vi "Filter Cluster Items.vi"(7 "Action":T1, 10 "Filter Str":string, 11 "Display Items":T2[](array[typedef])) -> (3 "Filtered Items":T2[](array[typedef]))   [LabVIEW 2023]
uses:
  cluster/Cluster Element Description.ctl
  controls/action enum.ctl
  <userlib>/_OpenG.lib/array/array.llb/Filter 1D Array with Scalar (I32)__ogtk.vi
  <userlib>/_OpenG.lib/array/array.llb/Remove Duplicates from 1D Array (I32)__ogtk.vi
  <userlib>/_OpenG.lib/array/array.llb/Index 1D Array Elements (Variant)__ogtk.vi
  <userlib>/_OpenG.lib/array/array.llb/openg_array.lvlib
panel:
  out "Array":cluster{"Array":string[]}[](array[cluster])
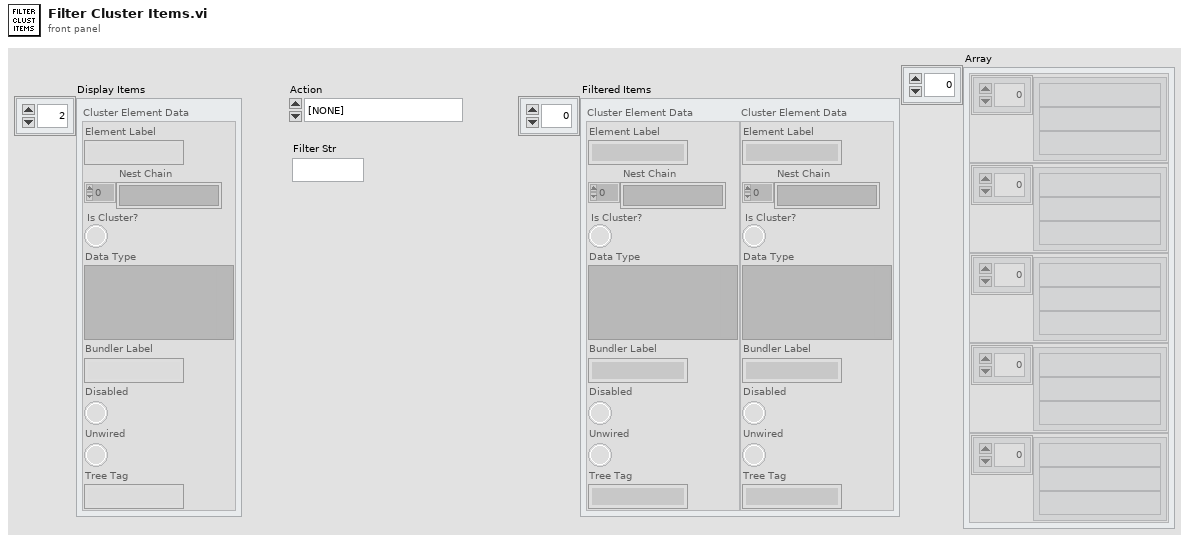
[diagram p1: front panel]
types:
  T1 = typedef "action enum.ctl" = enum16{"[NONE]", "APP_SEPARATOR", "Wire Bundle", "Wire Unbundle", "Terminal Unbundle", "Terminal Bundle", "Bundler Move Up", "Bundler Move Down", "Bundler Insert", "Bundler Remove", "Bundler Remove Unwired", "Bundler Rearrange", "In Place Insert", "In Place Remove", "In Place Remove Unwired", "In Place Rearrange", "Wire Properties", "Wire Method", "Terminal Properties", "Terminal Method", "Property Move Up", "Property Move Down", "Properties Insert", "Properties Remove", "Properties Remove Unwired", "Properties Rearrange", "Method Change", "Class For Constant", "Class For Control", "Class For Node", "Class Name to Clipboard"}
  T2 = typedef "Cluster Element Description.ctl" = cluster{"Element Label":string, "Nest Chain":string[], "Is Cluster?":bool, "Data Type":variant, "Bundler Label":string, "Disabled":bool, "Unwired":bool, "Tree Tag":string}
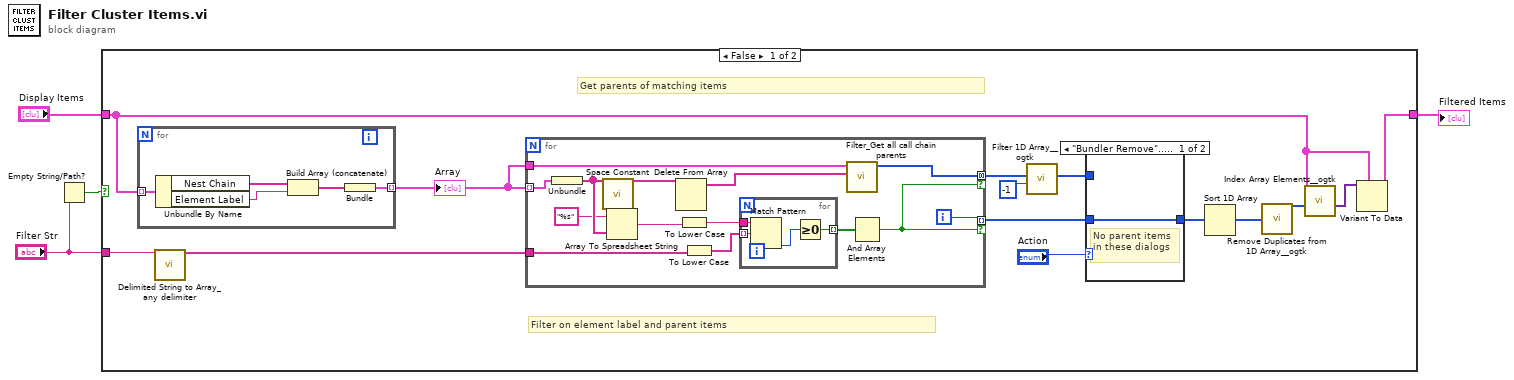
[diagram p0: block diagram]
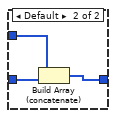
[diagram p2: hidden frame]
diagram:
  n1 = Empty String/Path?(string/path="Filter Str") -> (empty?=w1:bool)
  n2 = case shown="False" w1 {
    tunnel: [w9 w46] -> w4
    tunnel: "Display Items" -> [w8 w46]
    tunnel: "Filter Str" -> [w6 _]
    frame False {
      # "Filter on element label and parent items"
      # "Get parents of matching items"
      n3 = for {
        tunnel: w8 -> [w23] mode=indexing
        tunnel: [w19] -> w18 mode=indexing
        n4 = Unbundle By Name(w23) -> ("Nest Chain"=w22:string[], "Element Label"=w21:string)
        n5 = Build Array (concatenate)(w22, w21) -> (w20:string[])
        n6 = Bundle(w20) -> (w19:cluster{string[]})  [unwired: 1 in]
      }
      "Array" <- w18
      n7 = call "Delimited String to Array_any delimiter.vi"("Delimted String"=w6) -> ("Array"=w7:string[])  [unwired: 10 in]
      n8 = for {
        tunnel: w18 -> [w36] mode=indexing
        tunnel: w18 -> [w31]
        tunnel: [w41] -> w17 mode=indexing if=w28
        tunnel: [w29] -> w14 mode=concatenating if=w28
        tunnel: w7 -> [w37]
        i -> [w41]
        n9 = Unbundle(w36) -> (w35:string[])
        n10 = call <vilib>:"Space Constant.vi"() -> ("String"=w33:string)
        n11 = Array To Spreadsheet String(delimiter (Tab)=w33, array=w35, 3:"%s" ("format string")) -> (spreadsheet string=w32:string)
        n12 = Delete From Array(array=w35) -> (array with subset deleted=w30:string[])  [unwired: 2 in, 1 out]
        n13 = To Lower Case(string=w32) -> (all lower case string=w39:string)
        n14 = To Lower Case(string=w37) -> (all lower case string=w38:string[])
        n15 = for {
          tunnel: [w44] -> w40 mode=indexing
          tunnel: w39 -> [w43]
          tunnel: w38 -> [w42] mode=indexing
          n16 = Match Pattern(string=w43, regular expression=w42) -> (offset past match=w45:i32)  [unwired: 1 in, 3 out]
          n17 = Greater Or Equal To 0?(x=w45) -> (x >= 0?=w44:bool)
        }
        n18 = call "Filter_Get all call chain parents.vi"("Call Chain"=w30, "Array"=w31) -> ("parent indicies"=w29:i32[])  [unwired: 9 in]
        n19 = And Array Elements(Boolean array=w40) -> (logical AND=w28:bool)
      }
      n20 = call-poly <userlib>:"Filter 1D Array__ogtk.vi"("items to filter"=-1, "array"=w14) -> ("filtered array"=w12:i32[])  [unwired: 4 in, 1 out]
      n21 = case shown="\"Bundler Remove\"..\"Bundler Rearrange\"" "Action" {
        tunnel: w17 -> [w24 w27]
        tunnel: [w24 w26] -> w16
        tunnel: w12 -> [_ w25]
        frame "Bundler Remove".."Bundler Rearrange" {
          # "No parent items in these dialogs"
        }
        frame Default {
          n22 = Build Array (concatenate)(w25, w27) -> (w26:i32[])
        }
      }
      n23 = Sort 1D Array(array=w16) -> (sorted array=w15:i32[])
      n24 = call-poly <userlib>:"Remove Duplicates from 1D Array__ogtk.vi"("Input Array"=w15) -> ("Output Array"=w5:i32[])  [unwired: 1 out]
      n25 = call-poly <userlib>:"Index Array Elements__ogtk.vi"("indices"=w5, "array"=w8) -> ("elements"=w10:variant[])  [unwired: 9 in]
      n26 = Variant To Data(type=w8, Variant=w10) -> (data=w9:T2[])  [unwired: 1 in, 1 out]
    }
    frame True {
    }
  }
  "Filtered Items" <- w4
